vi "PumpCommand.vi"(7 "error in (no error)":errorcluster, 8 "Command:":string, 9 "Pump Address":enum16{"00", "01", "02", "03"}(ring), 10 "VISA Refnum in":refnum<visa-resource-name>) -> (0 "error out":errorcluster, 1 "EXIT PROGRAM? (F)":bool, 2 "Read (Response)":string, 3 "VISA resource name out":refnum<visa-resource-name>)   [LabVIEW 2014]
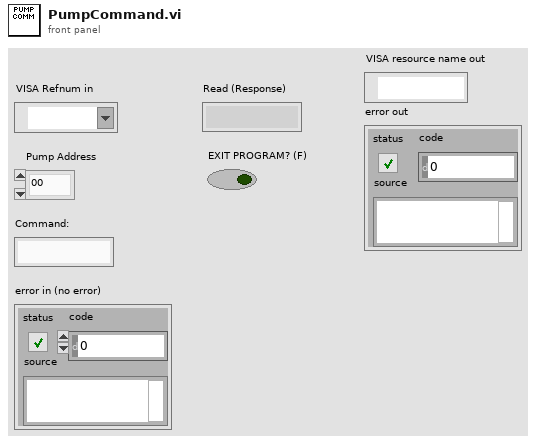
[diagram p1: front panel]
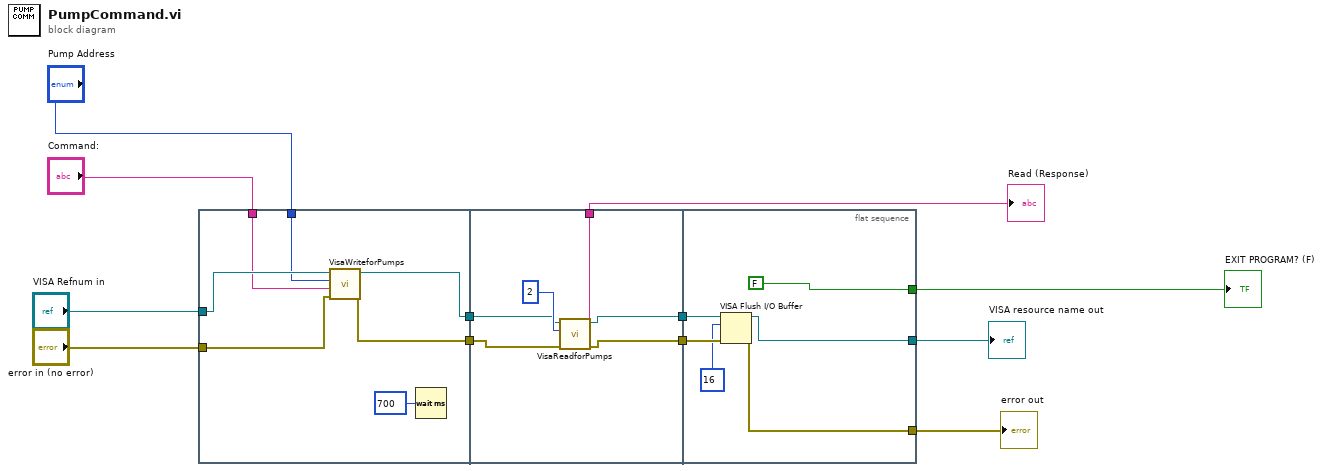
[diagram p0: block diagram]
diagram:
  n1 = flat-sequence {
    tunnel: [w17] -> w12
    tunnel: [w16] -> w11
    tunnel: "VISA Refnum in" -> [w19]
    tunnel: "error in (no error)" -> [w18]
    tunnel: "Pump Address" -> [w15]
    tunnel: "Command:" -> [w14]
    tunnel: [w22] -> w10
    tunnel: w12 -> [w23]
    tunnel: w11 -> [w24]
    tunnel: [w21] -> w9
    tunnel: [w20] -> w8
    tunnel: w10 -> [w31]
    tunnel: w9 -> [w30]
    tunnel: [FALSE] -> w5
    tunnel: [w27] -> w2
    tunnel: [w26] -> w1
    frame #0 {
      n2 = call "VisaWriteforPumps.vi"("error in (no error)"=w18, "Command:"=w14, "Pump Address"=w15, "VISA Refnum in"=w19) -> ("error out"=w16:errorcluster, "VISA Refnum out"=w17:refnum<visa-resource-name>)  [unwired: 6 in]
      n3 = Wait (ms)(milliseconds to wait=u32 700) -> ()  [unwired: 1 out]
    }
    frame #1 {
      n4 = call "VisaReadforPumps.vi"("error in (no error)"=w24, "Byte Count"=2, "VISA Refnum in"=w23) -> ("error out"=w21:errorcluster, "Read (Response)"=w20:string, "VISA Refnum out"=w22:refnum<visa-resource-name>)  [unwired: 5 in, 1 out]
    }
    frame #2 {
      n5 = VISA Flush I/O Buffer(VISA resource name=w31, mask (16)=16, error in (no error)=w30) -> (VISA resource name out=w27:refnum<visa-resource-name>, error out=w26:errorcluster)
    }
  }
  "Read (Response)" <- w8
  "EXIT PROGRAM? (F)" <- w5
  "VISA resource name out" <- w2
  "error out" <- w1
